vi "Write serialCommunicator.vi"(10 "serialCommunicator":refnum<class "SerialCommunicator.lvclass">, 11 "EncoderReader in":refnum<class "EncoderReader.lvclass">) -> (3 "EncoderReader out":refnum<class "EncoderReader.lvclass">)   [LabVIEW 2013, in "EncoderReader.lvlib" / "EncoderReader.lvclass"]
uses:
  <userlib>/Common/Devices/EncoderReader/EncoderReader/EncoderReader.lvclass
  <userlib>/Common/SerialProtocols/SerialCommunicator/SerialCommunicator.lvclass
  <userlib>/Common/Devices/EncoderReader/EncoderReader/EncoderReader.lvclass/EncoderReader.ctl
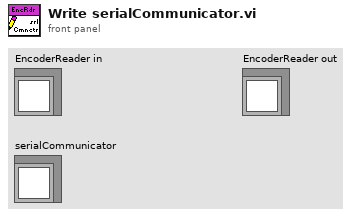
[diagram p1: front panel]
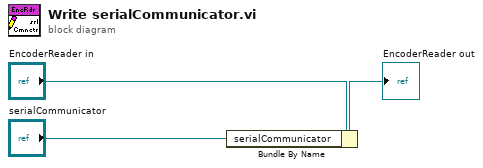
[diagram p0: block diagram]
diagram:
  n1 = Bundle By Name(cluster="EncoderReader in", "serialCommunicator"="serialCommunicator") -> (→"EncoderReader out":refnum<class "EncoderReader.lvclass">)
